vi "Get.vi"(8 "error in (no error)":errorcluster) -> (0 "error out":errorcluster, 3 "Master Reference":T1)   [LabVIEW 2017, in "SSH.lvlib" / "VI Reference Management.lvlib"]
doc: "Get the master reference for the cloneable Main VI.\n_____\nCreated using Delacor QMH Event Scripter 5.0.0.109."
uses:
  VI Reference Management.lvlib
  Main VI Type--strict_vi_ref.ctl
  builds/dqmh.lvlibp/1abvi3w/vi.lib/Delacor/Delacor QMH/Libraries/Cloneable Module Admin_class/Delacor_lib_QMH_Cloneable Module Admin.lvclass
  Action--enum.ctl
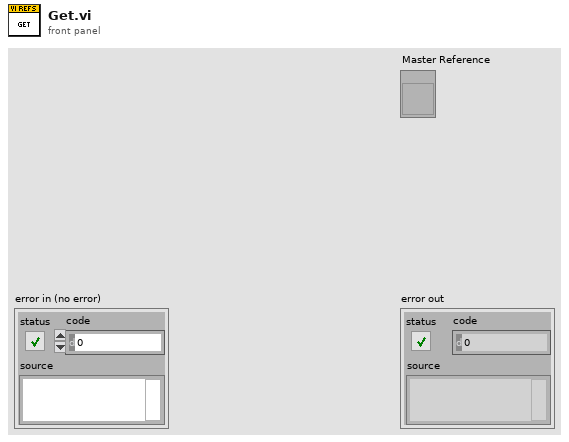
[diagram p1: front panel]
types:
  T1 = typedef "SSH.lvlib/VI Reference Management.lvlib/Main VI Type--strict_vi_ref.ctl" = refnum<vi>
  T2 = typedef "SSH.lvlib/VI Reference Management.lvlib/Action--enum.ctl" = enum16{"Get", "Create", "Close"}
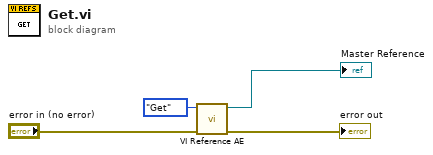
[diagram p0: block diagram]
diagram:
  n1 = call "VI Reference AE.vi"("error in (no error)"="error in (no error)", "Action"=Action--enum."Get") -> ("error out"=→"error out":errorcluster, "Master Reference"=→"Master Reference":T1)  [unwired: 7 in]
